vi "verify errors.vi"(8 "error in (no error)":errorcluster, 11 "Channel in":refnum<class "ECHARPE_Channel.lvclass">) -> (0 "error out":errorcluster, 2 "error":bool, 3 "Channel out":refnum<class "ECHARPE_Channel.lvclass">)   [LabVIEW 2018, in "ECHARPE_Channel.lvclass"]
uses:
  ECHARPE_Channel.lvclass
  Sim_CCD/Sim_CCD.lvclass/Sim_CCD.ctl
  Sim_CCD/Sim_CCD.lvclass
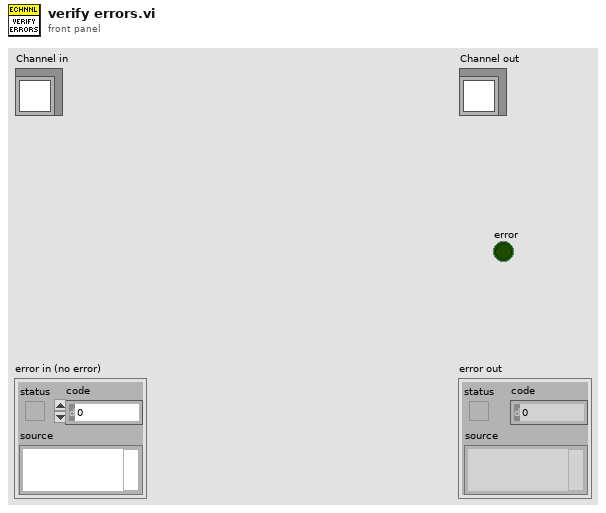
[diagram p1: front panel]
types:
  T1 = cluster{"#CYCLES":errorcluster, "SUFFIX":errorcluster}
  T2 = cluster{"State Machine.lvclass":refnum<class "State Machine.lvclass">, "RxTx.lvclass":refnum<class "RxTx.lvclass">, "Save_Header_RxTx.lvclass":refnum<class "RxTx.lvclass">, "Status SM.lvclass":refnum<class "State Machine.lvclass">, "Status RxTx.lvclass":refnum<class "RxTx.lvclass">, "servers array":refnum<class "Server.lvclass">[], "Events log file.lvclass":refnum<class "Log File.lvclass">, "Errors log file.lvclass":refnum<class "Log File.lvclass">, "Keywords log file.lvclass":refnum<class "Log File.lvclass">, "Sim_CCD.lvclass":refnum<class "Sim_CCD.lvclass">}
  T3 = cluster{"EXPTIME":errorcluster, "#FRAMES":errorcluster, "COOLER_POWER_STATUS":errorcluster, "TEMP":errorcluster}
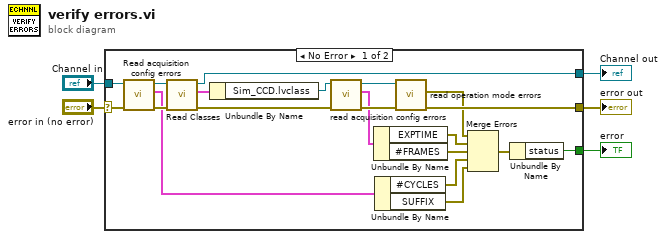
[diagram p0: block diagram]
diagram:
  n1 = case shown="No Error" "error in (no error)" {
    selector: "error in (no error)" -> [w10 w27]
    tunnel: [w23 w27] -> w4
    tunnel: [w13 w26] -> w2
    tunnel: "Channel in" -> [w12 w26]
    tunnel: [w21 _] -> w1
    frame No Error {
      n2 = call-dynamic "Read acquisition config errors.vi"("error in (no error)"=w10, "Channel in"=w12) -> ("error out"=w9:errorcluster, "acquisition config errors"=w8:T1, "Channel out"=w11:refnum<class "ECHARPE_Channel.lvclass">)  [unwired: 7 in]
      n3 = call-dynamic "Read Classes.vi"("error in (no error)"=w9, "Channel in"=w11) -> ("error out"=w14:errorcluster, "Classes"=w16:T2, "Channel out"=w13:refnum<class "ECHARPE_Channel.lvclass">)  [unwired: 7 in]
      n4 = Unbundle By Name(w16) -> ("Sim_CCD.lvclass"=w15:refnum<class "Sim_CCD.lvclass">)
      n5 = call "read acquisition config errors.vi"("error in (no error)"=w14, "Simulated Camera in"=w15) -> ("error out"=w25:errorcluster, "acquisition config errors"=w19:T3, "Simulated Camera out"=w24:refnum<class "Sim_CCD.lvclass">)  [unwired: 7 in]
      n6 = Unbundle By Name(w19) -> ("EXPTIME"=w18:errorcluster, "#FRAMES"=w17:errorcluster)
      n7 = Unbundle By Name(w8) -> ("#CYCLES"=w7:errorcluster, "SUFFIX"=w6:errorcluster)
      n8 = call "read operation mode errors.vi"("error in (no error)"=w25, "Simulated_CCD_Camera in"=w24) -> ("error out"=w23:errorcluster, "WRITE SETUP errors"=w20:errorcluster[])  [unwired: 7 in, 1 out]
      n9 = Merge Errors(w20, w18, w17, w7, w6) -> (w22:errorcluster)
      n10 = Unbundle By Name(w22) -> ("status"=w21:bool)
    }
    frame Error {
    }
  }
  "error out" <- w4
  "Channel out" <- w2
  "error" <- w1
